vi "filter.vi"(1 "输入数组":dbl[](array[numeric])) -> (0 "输出数组":dbl[](array[numeric]))   [LabVIEW 2018]
panel:
  out "h数组索引":dbl
  out "输入数组索引":dbl
  out "sum":dbl
  in  "h":dbl[](array[numeric]) format="%.16g"
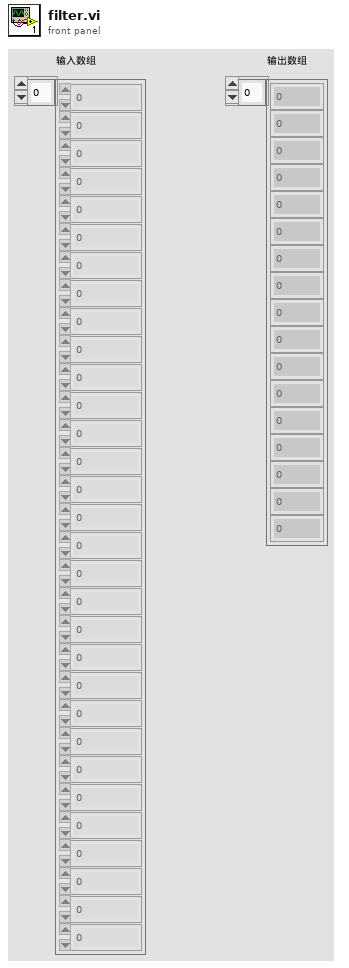
[diagram p1: front panel]
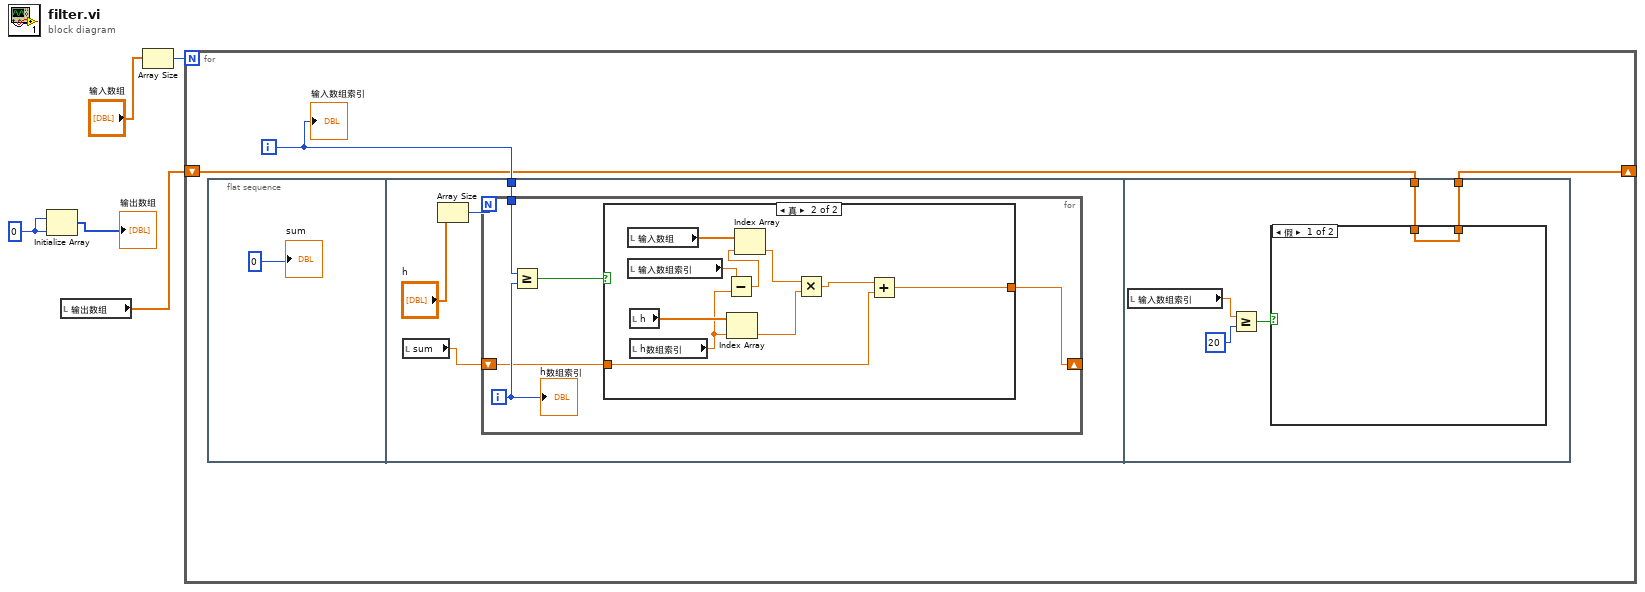
[diagram p0: block diagram]
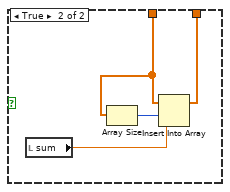
[diagram p3: hidden frame]
diagram:
  w2 = 0
  n1 = Initialize Array(w2, w2) -> (→"输出数组":i32[])
  n2 = local read "输出数组"() -> (w1:dbl[])
  n3 = Array Size(array="输入数组") -> (size(s)=w4:i32)
  n4 = for {
    N: w4 -> [_]
    shift-right: [w6] -> _
    shift-left: w1 -> [w7]
    i -> [w8]
    n5 = flat-sequence {
      tunnel: w8 -> [w11]
      tunnel: w7 -> [w31]
      tunnel: [w30] -> w6
      frame #0 {
        "sum" <- 0
      }
      frame #1 {
        n6 = local read "sum"() -> (w10:dbl)
        n7 = Array Size(array="h") -> (size(s)=w13:i32)
        n8 = for {
          N: w13 -> [_]
          tunnel: w11 -> [w18]
          shift-right: [w14] -> _
          shift-left: w10 -> [w15]
          i -> [w16]
          n9 = Greater Or Equal?(x=w18, y=w16) -> (x >= y?=w17:bool)
          n10 = case shown="真" w17 {
            tunnel: w15 -> [w19 w21]
            tunnel: [w19 w20] -> w14
            frame False {
            }
            frame True {
              n11 = local read "输入数组"() -> (w28:dbl[])
              n12 = local read "输入数组索引"() -> (w26:dbl)
              n13 = local read "h"() -> (w29:dbl[])
              n14 = local read "h数组索引"() -> (w25:dbl)
              n15 = Subtract(x=w26, y=w25) -> (x-y=w27:dbl)
              n16 = Index Array(array=w29, index=w25) -> (element=w23:dbl)
              n17 = Index Array(array=w28, index=w27) -> (element=w24:dbl)
              n18 = Multiply(x=w24, y=w23) -> (x*y=w22:dbl)
              n19 = Add(x=w22, y=w21) -> (x+y=w20:dbl)
            }
          }
          "h数组索引" <- w16
        }
      }
      frame #2 {
        n20 = local read "输入数组索引"() -> (w33:dbl)
        n21 = Greater Or Equal?(x=w33, y=20) -> (x >= y?=w32:bool)
        n22 = case shown="假" w32 {
          tunnel: w31 -> [w35 w37]
          tunnel: [w35 w36] -> w30
          frame False {
          }
          frame True {
            n23 = local read "sum"() -> (w39:dbl)
            n24 = Array Size(array=w37) -> (size(s)=w38:i32)
            n25 = Insert Into Array(array=w37, index=w38, new element=w39) -> (w36:dbl[])
          }
        }
      }
    }
    "输入数组索引" <- w8
  }
